vi "GetPeak.vi"(8 "error in (no error)":errorcluster, 11 "Instruments in":refnum<class "Instruments.lvclass">) -> (0 "error out":errorcluster, 2 "Peak Wl":dbl, 3 "Instruments out":refnum<class "Instruments.lvclass">)   [LabVIEW 2012, in "Instruments.lvclass"]
uses:
  Instruments.lvclass
  Instruments.lvclass/Instruments.ctl
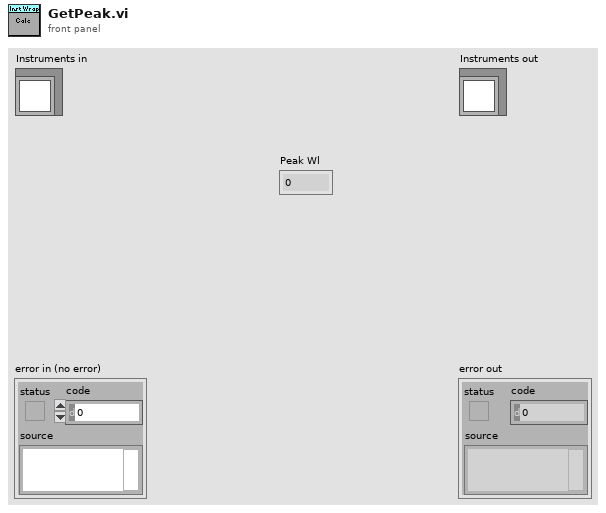
[diagram p1: front panel]
types:
  T1 = typedef "SMUParam.ctl" = cluster{"Start Current,mA":dbl, "Stop Current,mA":dbl, "Voltage Compliance,V":dbl, "GPIB":string, "VISA resource name":refnum<visa-resource-name>}
  T2 = typedef "USB4000_Data.ctl" = cluster{"Wrapper Out":u32, "Number of Spectrometers":i32, "Wavelength":dbl[], "EL Spectrum":dbl[], "Int Time (usec)":i32, bool, "Background":dbl[]}
  T3 = typedef "OphirRef.ctl" = cluster{"OphirComRef":refnum<k7>, "deviceHandle":i32, "Channel":i32, "SerialNumber":string, "Background Wl":dbl, "Background":dbl, "CalWl":dbl}
  T4 = typedef "Config.ctl" = cluster{"IntTime":i32, "Samples":i32, "PowerMin":dbl, "KneeMin":dbl, "KneeMax":dbl, "Background Wl":dbl, "Settle Delay,ms":u32, "StationId":sgl}
  T5 = cluster{"Keithley_Param":T1, "USB4000_Param":cluster{"Integration Time":i32, "Wl min,nm":dbl, "Wl max,nm":dbl, "USB4000":T2}, "OphirCntrlRef":T3, "Config":T4}
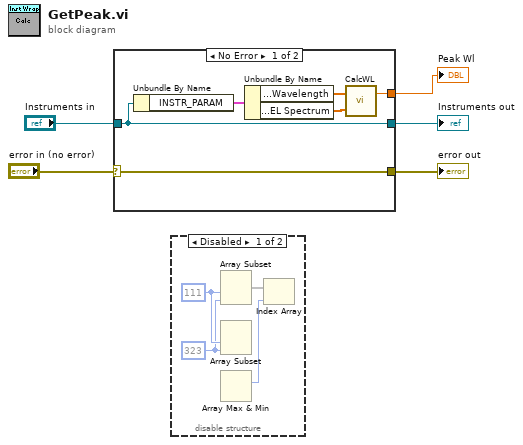
[diagram p0: block diagram]
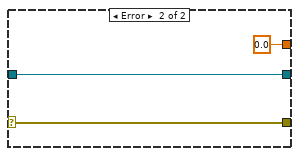
[diagram p3: hidden frame]
diagram:
  n1 = case shown="No Error" "error in (no error)" {
    selector: "error in (no error)" -> [w11 w14]
    tunnel: [w11 w14] -> w4
    tunnel: [w10 w13] -> w2
    tunnel: "Instruments in" -> [w10 w13]
    tunnel: [w6 0.0] -> w1
    frame No Error {
      n2 = Unbundle By Name(w10) -> ("INSTR_PARAM"=w9:T5)
      n3 = Unbundle By Name(w9) -> ("USB4000_Param.USB4000.Wavelength"=w8:dbl[], "USB4000_Param.USB4000.EL Spectrum"=w7:dbl[])
      n4 = call "CalcWL.vi"("Spectra"=w7, "Lambda"=w8) -> ("Peak WL"=w6:dbl)  [unwired: 1 out]
    }
    frame Error {
    }
  }
  "error out" <- w4
  "Instruments out" <- w2
  "Peak Wl" <- w1
  n5 = disable-structure shown="Disabled" {
    frame Disabled {
      w18 = 111 ("index")
      w17 = 323 ("length")
      n6 = Array Subset(index=w18, length=w17) -> (w15:void[])  [unwired: 1 in]
      n7 = Array Subset(index=w18, length=w17) -> ()  [unwired: 1 in, 1 out]
      n8 = Array Max & Min() -> (max index (indices)=w16:i32)  [unwired: 1 in, 3 out]
      n9 = Index Array(array=w15, index=w16) -> ()  [unwired: 1 out]
    }
    frame Enabled {
    }
  }
